vi "ArdnoFlushFeed.vi"(0 "LINX Resource":T2={"IO"=enum."Remote", "Interface"=enum."Serial", "LINX Device Config"={"Interface"=enum."Serial", "COM Port"="COM13", "TCP Configuration"={"IP Address"="", "Port"=0}, "Device Family"=1, "Device ID"=1, "Device Name"="myRIO-1900", "TCP Ref"=refnum, "Channels"={"DI"=[0, 1, 2, 3, 4, 5, 6, 7, 8, 9, 10, 11, 12, 13, 14, 15, 16, 17, 18, 19, 20, 21, 22, 23, 24, 25, 26, 27, 28, 29, 30, 31, 32, 33, 34, 35, 36, 37, 38, 39, 40, 41, 42, 43, 44, 45, 46], "DO"=[0, 1, 2, 3, 4, 5, 6, 7, 8, 9, 10, 11, 12, 13, 14, 15, 16, 17, 18, 19, 20, 21, 22, 23, 24, 25, 26, 27, 28, 29, 30, 31, 32, 33, 34, 35, 36, 37, 38, 39, 40, 41, 42, 43, 44, 45, 46], "AI"=[0, 1, 2, 3, 4, 5, 6, 7, 8, 9, 10, 11], "AO"=[], "PWM"=[3, 5, 6, 9, 10], "QE"=[], "UART"=[0, 1], "I2C 2"=[0], "SPI"=[0], "CAN"=[], "Servo"=[], "AI Ref (V)"=0.0, "AI Resolution (Bits)"=0, "AO Ref (V)"=0.0, "AO Resolution (Bits)"=0}}}, 1 "Reagent":u32, 4 "Feed Cycles":i32, 5 "error in (no error)":errorcluster, 6 "Single / Multiring?":u16(ring) items=["8-Ring", "OneRing", "valveGR"]) -> (13 "ValveStates":bool[](array[boolean]), 14 "LINX Resource out":T2, 15 "Elapsed [ms]":u32, 19 "error out":errorcluster)   [LabVIEW 2018, in "Arduino.lvlib"]
uses:
  Arduino.lvlib
  <vilib>/MakerHub/LINX/Private/Type Defs/LINX Ref.ctl
  <vilib>/MakerHub/LINX/Private/Type Defs/Platform.ctl
  <vilib>/MakerHub/LINX/Private/Type Defs/Interface.ctl
  <vilib>/MakerHub/LINX/Private/Device/Type Defs/LINX Device Config.ctl
  <vilib>/MakerHub/LINX/Private/Device/Type Defs/TCP Config.ctl
  <vilib>/MakerHub/LINX/Private/Device/Type Defs/Channels.ctl
  <vilib>/MakerHub/LINX/Public/Peripherals/Digital/Digital Write N Chans.vi
  <vilib>/MakerHub/LINX/Private/Local IO/LinxDigitalWrite.vi
  <vilib>/MakerHub/LINX/Public/Utilities/Check Channel.vi
  <vilib>/MakerHub/LINX/Private/Utilties/Generate Error.vi
  <vilib>/MakerHub/LINX/LMH-LINX.lvlib
  <vilib>/MakerHub/LINX/Private/Device/Device.lvlib
panel:
  in  "ValveManualCluster":T1
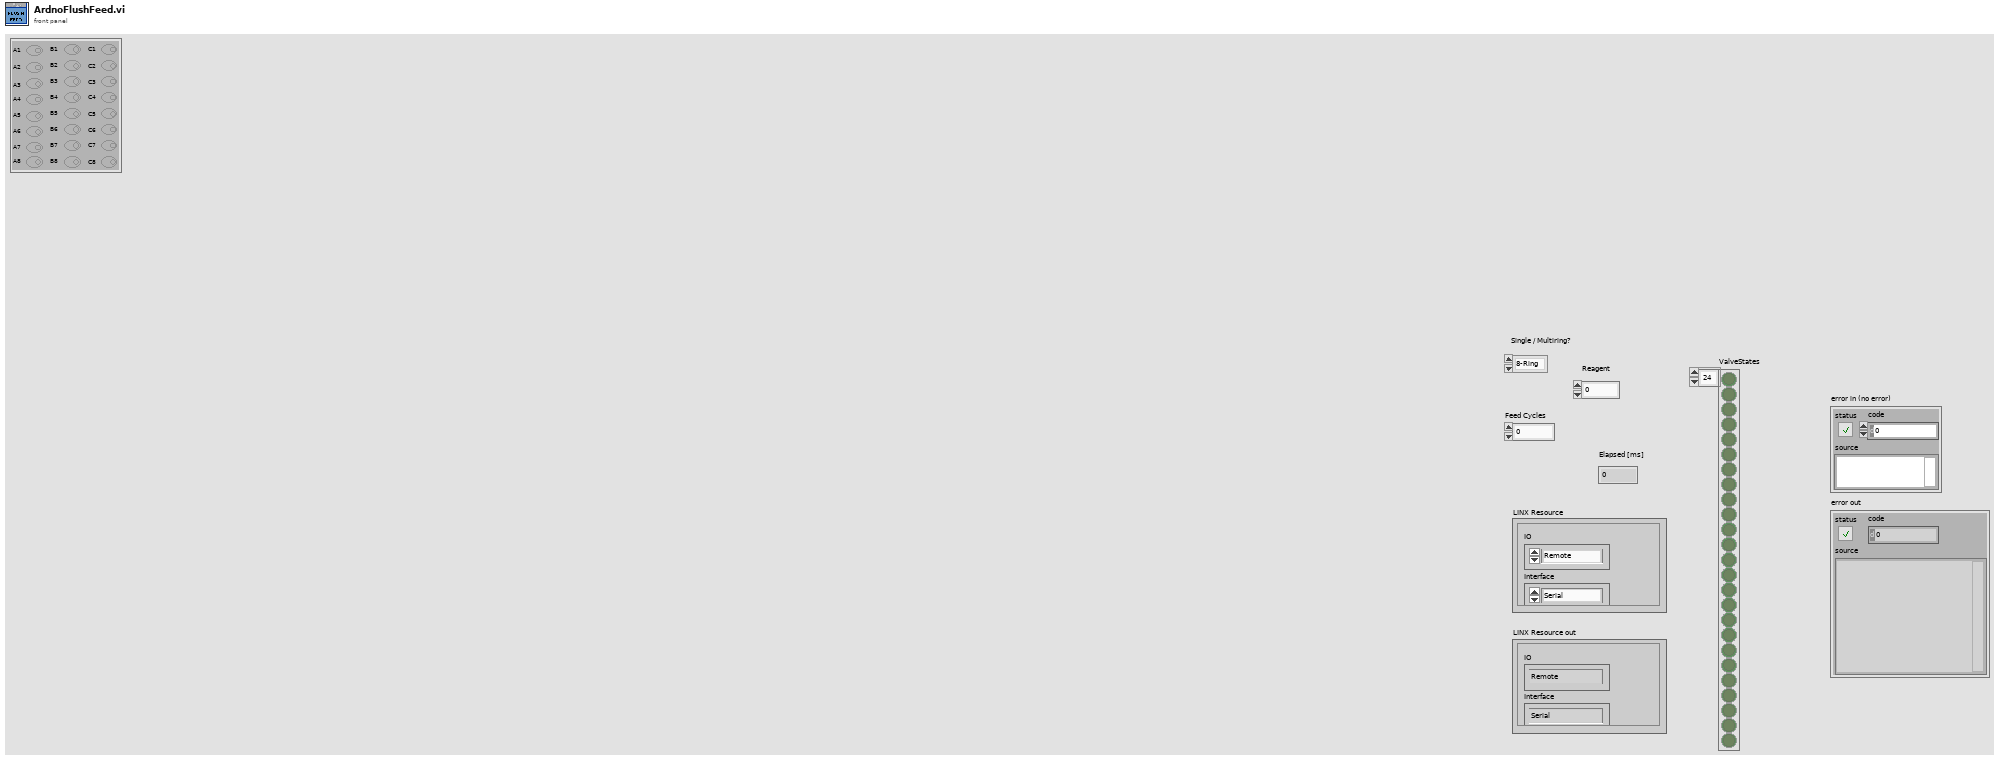
[diagram p1: front panel]
types:
  T1 = cluster{"C8":bool, "C7":bool, "C6":bool, "C5":bool, "C4":bool, "C3":bool, "C2":bool, "C1":bool, "B8":bool, "B7":bool, "B6":bool, "B5":bool, "B4":bool, "B3":bool, "B2":bool, "B1":bool, "A8":bool, "A7":bool, "A6":bool, "A5":bool, "A4":bool, "A3":bool, "A2":bool, "A1":bool}
  T2 = typedef "LMH-LINX.lvlib/LINX Ref.ctl" = cluster{"IO":T3, "Interface":T4, "LINX Device Config":T5}
  T3 = typedef "LMH-LINX.lvlib/Platform.ctl" = enum16{"Remote", "Local"}
  T4 = typedef "LMH-LINX.lvlib/Interface.ctl" = enum16{"Serial", "TCP"}
  T5 = typedef "LMH-LINX.lvlib/Device.lvlib/LINX Device Config.ctl" = cluster{"Interface":T4, "COM Port":refnum<visa-resource-name>, "TCP Configuration":T6, "Device Family":u8, "Device ID":u8, "Device Name":string, "TCP Ref":refnum<k5>, "Channels":T7}
  T6 = typedef "LMH-LINX.lvlib/Device.lvlib/TCP Config.ctl" = cluster{"IP Address":string, "Port":u16}
  T7 = typedef "LMH-LINX.lvlib/Channels.ctl" = cluster{"DI":u8[], "DO":u8[], "AI":u8[], "AO":u8[], "PWM":u8[], "QE":u8[], "UART":u8[], "I2C 2":u8[], "SPI":u8[], "CAN":u8[], "Servo":u8[], "AI Ref (V)":dbl, "AI Resolution (Bits)":u8, "AO Ref (V)":dbl, "AO Resolution (Bits)":u8}
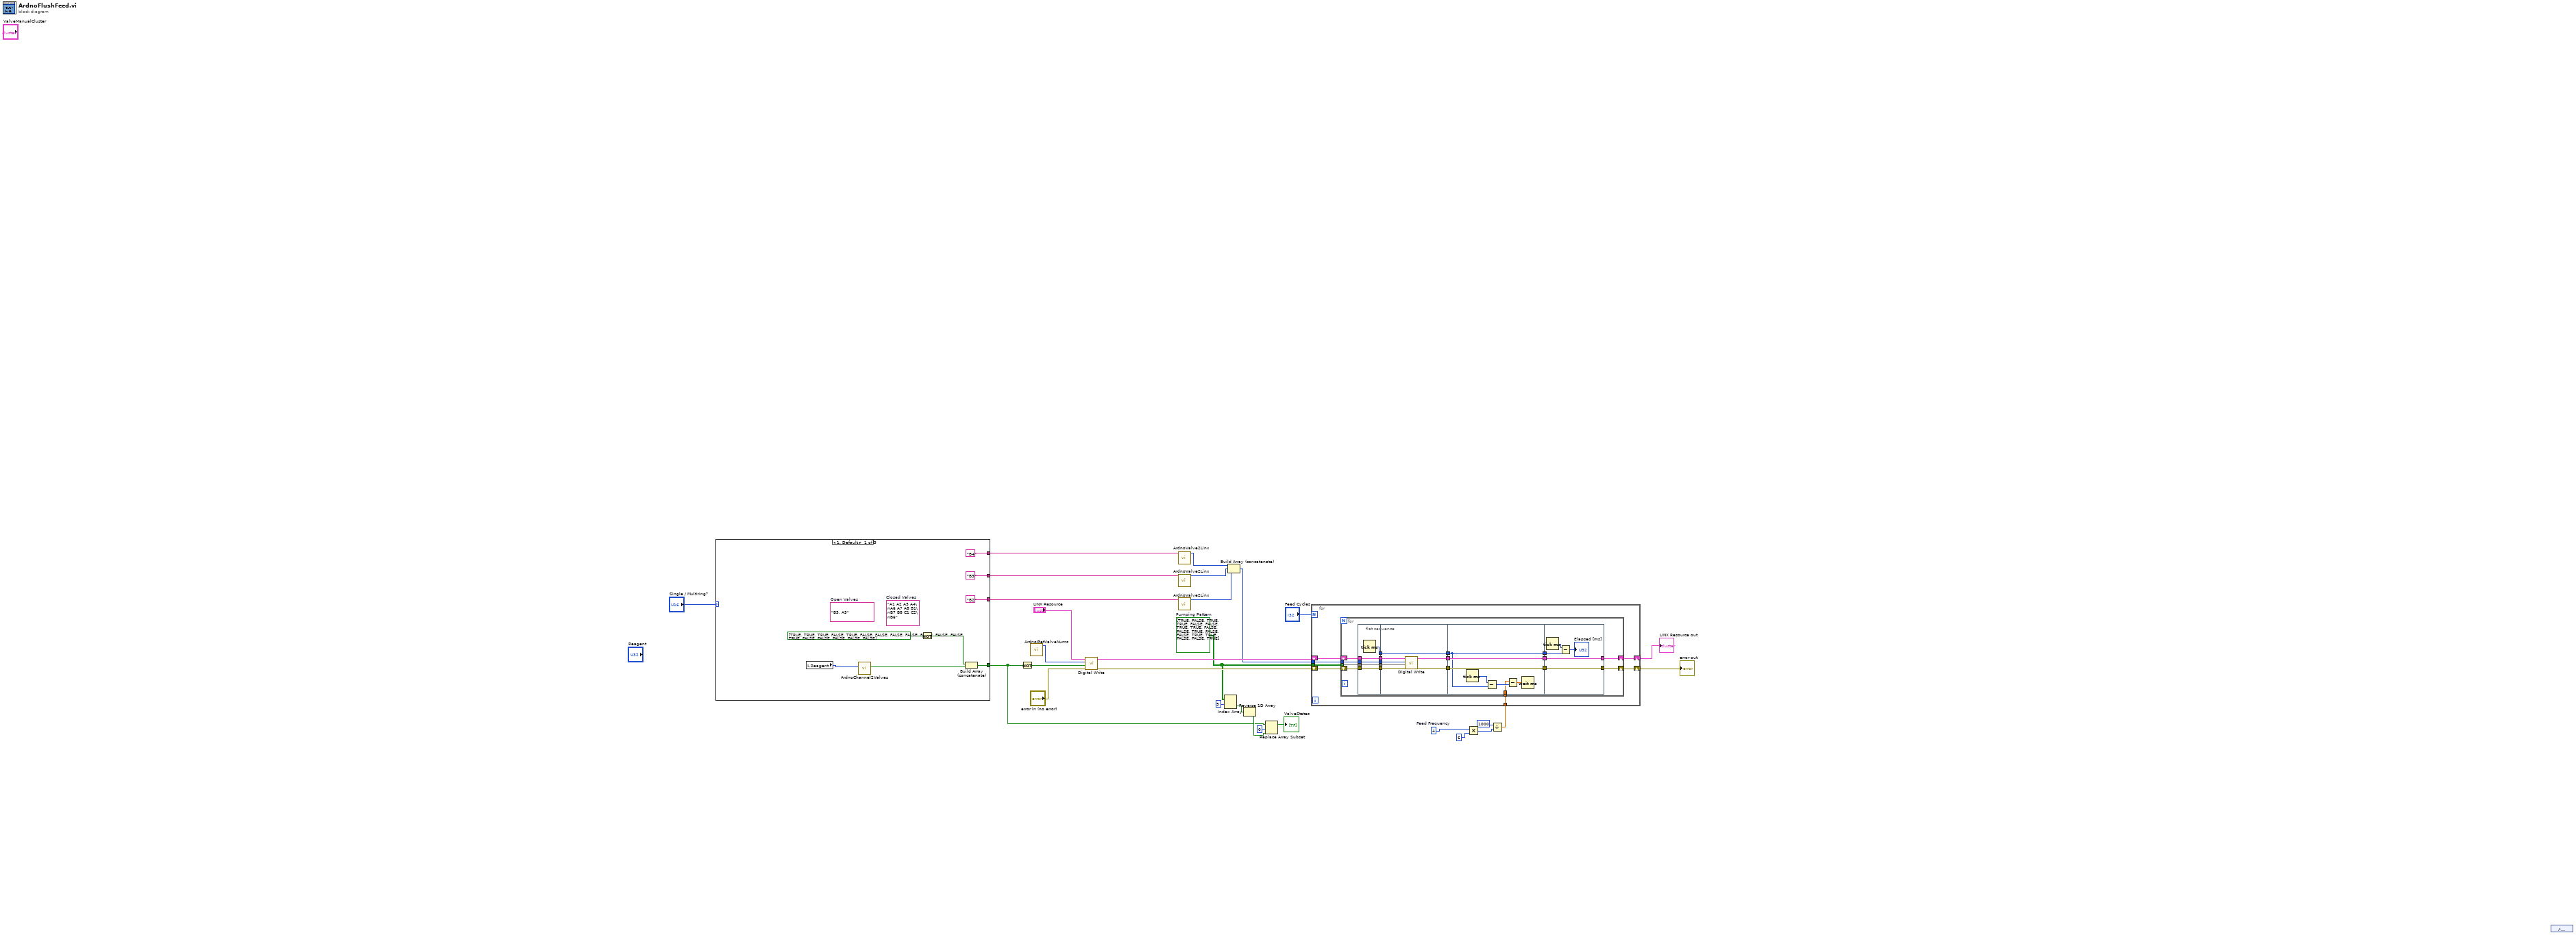
[diagram p0: block diagram]
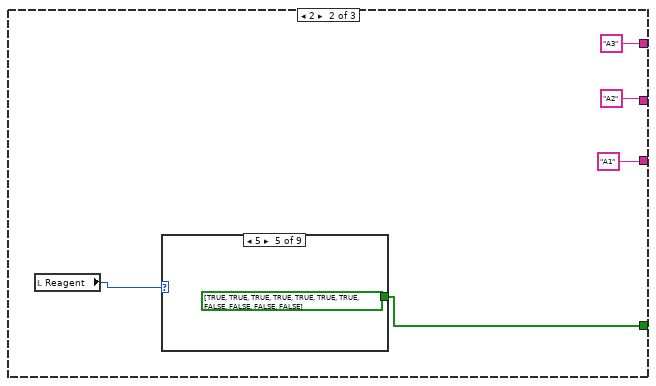
[diagram p2: hidden frame]
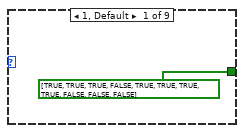
[diagram p3: hidden frame]
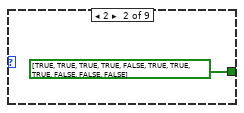
[diagram p4: hidden frame]
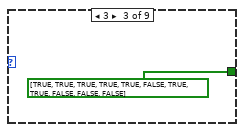
[diagram p5: hidden frame]
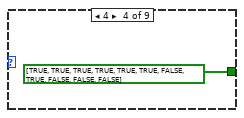
[diagram p6: hidden frame]
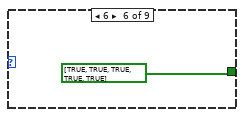
[diagram p7: hidden frame]
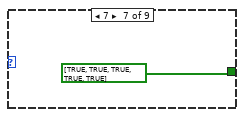
[diagram p8: hidden frame]
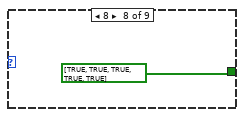
[diagram p9: hidden frame]
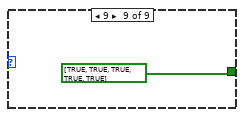
[diagram p10: hidden frame]
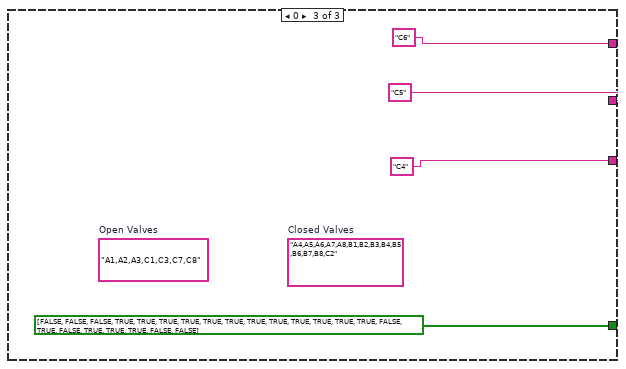
[diagram p11: hidden frame]
diagram:
  w19 = u32 4  # Feed Frequency
  w5 = bool[][] [[TRUE, FALSE, TRUE], [TRUE, FALSE, FALSE], [TRUE, TRUE, FALSE], [FALSE, TRUE, FALSE], [FALSE, TRUE, TRUE], [FALSE, FALSE, TRUE]]  # Pumping Pattern
  n1 = case shown="1, Default" "Single / Multiring?" {
    tunnel: [w34 w38 bool[] [FALSE, FALSE, FALSE, TRUE, TRUE, TRUE, TRUE, TRUE, TRUE, TRUE, TRUE, TRUE, TRUE, TRUE, TRUE, FALSE, TRUE, FALSE, TRUE, TRUE, TRUE, FALSE, FALSE]] -> w4
    tunnel: ["B2" "A1" "C4"] -> w12
    tunnel: ["B3" "A2" "C5"] -> w11
    tunnel: ["B4" "A3" "C6"] -> w10
    frame 1, Default {
      (unwired) "A1 A2 A3 A4\nA6 A7 A8 B1\nB7 B8 C1 C2\nB6"  # Closed Valves
      (unwired) "B5, A5"  # Open Valves
      n2 = local read "Reagent"() -> (w30:u32)
      n3 = call "ArdnoChannel2Valves.vi"("Reagent"=w30) -> ("Valve State"=w33:bool[])  [unwired: 9 in]
      n4 = Not(x=bool[] [TRUE, TRUE, TRUE, FALSE, TRUE, FALSE, FALSE, FALSE, FALSE, FALSE, FALSE, FALSE, TRUE, FALSE, FALSE, FALSE, FALSE, FALSE]) -> (.not. x?=w31:bool[])
      n5 = Build Array (concatenate)(w31, w33) -> (w34:bool[])
    }
    frame 2 {
      n6 = local read "Reagent"() -> (w39:u32)
      n7 = case shown="5" w39 {
        tunnel: [bool[] [TRUE, TRUE, TRUE, FALSE, TRUE, TRUE, TRUE, TRUE, FALSE, FALSE, FALSE] bool[] [TRUE, TRUE, TRUE, TRUE, FALSE, TRUE, TRUE, TRUE, FALSE, FALSE, FALSE] bool[] [TRUE, TRUE, TRUE, TRUE, TRUE, FALSE, TRUE, TRUE, FALSE, FALSE, FALSE] bool[] [TRUE, TRUE, TRUE, TRUE, TRUE, TRUE, FALSE, TRUE, FALSE, FALSE, FALSE] bool[] [TRUE, TRUE, TRUE, TRUE, TRUE, TRUE, TRUE, FALSE, FALSE, FALSE, FALSE] bool[] [TRUE, TRUE, TRUE, TRUE, TRUE] bool[] [TRUE, TRUE, TRUE, TRUE, TRUE] bool[] [TRUE, TRUE, TRUE, TRUE, TRUE] bool[] [TRUE, TRUE, TRUE, TRUE, TRUE]] -> w38
        frame 1, Default {
        }
        frame 2 {
        }
        frame 3 {
        }
        frame 4 {
        }
        frame 5 {
        }
        frame 6 {
        }
        frame 7 {
        }
        frame 8 {
        }
        frame 9 {
        }
      }
    }
    frame 0 {
      (unwired) "A4,A5,A6,A7,A8,B1,B2,B3,B4,B5,B6,B7,B8,C2"  # Closed Valves
      (unwired) "A1,A2,A3,C1,C3,C7,C8"  # Open Valves
    }
  }
  n8 = Not(x=w4) -> (.not. x?=w1:bool[])
  n9 = call "ArdnoGetValveNums.vi"() -> ("Array"=w2:i32[])  [unwired: 11 in]
  n10 = call-poly <vilib>:"Digital Write.vi"("Error In"="error in (no error)", "Values"=w1, "DO Channels"=w2, "LINX Resource"="LINX Resource") -> ("Error Out"=w24:errorcluster, "LINX Resource"=w23:T2)  [unwired: 6 in]
  n11 = call "ArdnoValve2Linx.vi"("Valve (A1-C8),\n comma separated"=w10) -> ("Linx Port"=w13:i32[])  [unwired: 8 in, 2 out]
  n12 = call "ArdnoValve2Linx.vi"("Valve (A1-C8),\n comma separated"=w11) -> ("Linx Port"=w14:i32[])  [unwired: 8 in, 2 out]
  n13 = call "ArdnoValve2Linx.vi"("Valve (A1-C8),\n comma separated"=w12) -> ("Linx Port"=w15:i32[])  [unwired: 8 in, 2 out]
  n14 = Index Array(array=w5, index (row)=5) -> (element=w8:bool[])  [unwired: 1 in]
  n15 = Build Array (concatenate)(w13, w14, w15) -> (w18:i32[])
  n16 = Reverse 1D Array(array=w8) -> (reversed array=w7:bool[])
  n17 = Replace Array Subset(array=w4, new element=w7, index=0) -> (→"ValveStates":bool[])
  n18 = Multiply(x=w19, y=u32 6) -> (x*y=w25:u32)
  n19 = Divide(x=u32 1000, y=w25) -> (x/y=w26:dbl)
  n20 = for {
    N: "Feed Cycles" -> [_]
    tunnel: w18 -> [w60]
    tunnel: w5 -> [w59]
    shift-right: [w58] -> w22
    shift-left: w23 -> [w62]
    shift-right: [w57] -> w21
    shift-left: w24 -> [w61]
    tunnel: w26 -> [w56]
    n21 = for {
      tunnel: w59 -> [w75] mode=indexing
      tunnel: w60 -> [w78]
      shift-right: [w77] -> w58
      shift-left: w62 -> [w80]
      shift-right: [w76] -> w57
      shift-left: w61 -> [w79]
      tunnel: w56 -> [w66]
      n22 = flat-sequence {
        tunnel: w75 -> [w82]
        tunnel: w78 -> [w83]
        tunnel: w79 -> [w84]
        tunnel: w80 -> [w85]
        tunnel: [w85] -> w74
        tunnel: [w84] -> w73
        tunnel: [w83] -> w72
        tunnel: [w82] -> w71
        tunnel: [w81] -> w70
        tunnel: [w89] -> w65
        tunnel: [w88] -> w64
        tunnel: w74 -> [w92]
        tunnel: w73 -> [w91]
        tunnel: w72 -> [w90]
        tunnel: w71 -> [w87]
        tunnel: w70 -> [w86]
        tunnel: [w86] -> w63
        tunnel: w65 -> [w99]
        tunnel: w64 -> [w98]
        tunnel: w63 -> [w96]
        tunnel: [w99] -> w69
        tunnel: [w98] -> w68
        tunnel: [w96] -> w67
        tunnel: w66 -> [w93]
        tunnel: [w103] -> w76
        tunnel: [w104] -> w77
        tunnel: w69 -> [w104]
        tunnel: w68 -> [w103]
        tunnel: w67 -> [w100]
        frame #0 {
          n23 = Tick Count (ms)() -> (millisecond timer value=w81:u32)
        }
        frame #1 {
          n24 = call-poly <vilib>:"Digital Write.vi"("Error In"=w91, "Values"=w87, "DO Channels"=w90, "LINX Resource"=w92) -> ("Error Out"=w88:errorcluster, "LINX Resource"=w89:T2)  [unwired: 6 in]
        }
        frame #2 {
          n25 = Tick Count (ms)() -> (millisecond timer value=w97:u32)
          n26 = Subtract(x=w97, y=w96) -> (x-y=w95:u32)
          n27 = Subtract(x=w93, y=w95) -> (x-y=w94:dbl)
          n28 = Wait (ms)(milliseconds to wait=w94) -> ()  [unwired: 1 out]
        }
        frame #3 {
          n29 = Tick Count (ms)() -> (millisecond timer value=w101:u32)
          n30 = Subtract(x=w101, y=w100) -> (x-y=→"Elapsed [ms]":u32)
        }
      }
    }
  }
  "error out" <- w21
  "LINX Resource out" <- w22
  n31 = control-ref of="ValveManualCluster"() -> ()  [unwired: 1 out]
